vi "DFT_Update Spectra.vi"(6 "averages completed":dbl, 9 "spectra info":T1[](array[typedef]) {"x-axis units" items=["Time (s)"=0, "Frequency-CB (Hz)"=1, "Frequency-CPB (Hz)"=1248, "Frequency-Arbitrary (Hz)"=2357, "Quefrency (s)"=2, "Revolutions (rev)"=3, "Order"=4, "Speed (RPM)"=11, "Speed (rad/s)"=21, "Index"=65535]; "weighting filter" items=["Linear", "A-weighting", "B-weighting", "C-weighting", "ITU-R 468-4", "Dolby", "CCITT", "C-message", "Wb", "Wc", "Wd", "We", "Wf", "Wh", "Wj", "Wk", "Wm", "AES17 20 kHz lowpass", "AES17 40 kHz lowpass", "AES17 20 kHz highpass", "AES17 40 kHz highpass"]; "dB reference [EU]" format="%.2f"; "engineering units" items=["custom..."=0, "V"=1, "A"=21, "C"=30, "pC"=31, "s"=32, "-"=29, "Pa"=2, "N"=20, "g"=3, "m/s^2"=4, "m/s"=5, "m"=6, "mm/s"=12, "mm"=13, "micron/s"=14, "micron"=15, "in/s^2"=7, "in/s"=8, "in"=9, "mil/s"=10, "mil"=11, "rad/s^2"=16, "rad/s"=17, "rad"=18, "deg/s^2"=26, "deg/s"=27, "deg"=28, "RPM"=22, "cycle/s^2"=23, "Hz"=24, "cycle"=25, "strain"=19]; "spectral info"."window" items=["None "=0, "Hanning"=1, "Hamming"=2, "Blackman-Harris"=3, "Exact Blackman"=4, "Blackman"=5, "Flat Top"=6, "4 Term B-Harris "=7, "7 Term B-Harris"=8, "Low Sidelobe"=9, "Force - Exponential"=10, "Gaussian"=62]}, 10 "spectra":cluster{"f0":dbl, "df":dbl, "magnitude":dbl[]}[](array[cluster]) {"magnitude" format="%.2p"; "df" format="%.2p"; "f0" format="%.2p"}, 11 "Data":T7={"First Time"=FALSE, "Show Results Window"=FALSE, "Show Results Window Clicked"=FALSE, "Window"=1, "overlap"=50, "Block Duration"=0.1, "Averaging parameters"={"averaging mode"=enum."No averaging", "weighting mode"=enum."Exponential", "number of averages"=10}, "buffer out"=refnum, "Avg Spectra"=refnum, "Spectra UI"=refnum} {"Averaging parameters"."number of averages" min=1; "Window" items=["Rectangle"=0, "Hanning"=1, "Hamming"=2, "Blackman-Harris"=3, "Exact Blackman"=4, "Blackman"=5, "Flat Top"=6, "4 Term B-Harris "=7, "7 Term B-Harris"=8, "Low Sidelobe"=9, "Blackman Nuttall"=11, "Triangle"=30, "Bartlett-Hanning"=31, "Bohman"=32, "Parzen"=33, "Welch"=34, "Kaiser"=60, "Dolph-Chebyshev"=61, "Gaussian"=62]}) -> (3 "Data out":T7={"First Time"=FALSE, "Show Results Window"=FALSE, "Show Results Window Clicked"=FALSE, "Window"=1, "overlap"=50, "Block Duration"=0.1, "Averaging parameters"={"averaging mode"=enum."No averaging", "weighting mode"=enum."Exponential", "number of averages"=10}, "buffer out"=refnum, "Avg Spectra"=refnum, "Spectra UI"=refnum} {"Averaging parameters"."number of averages" min=1; "Window" items=["Rectangle"=0, "Hanning"=1, "Hamming"=2, "Blackman-Harris"=3, "Exact Blackman"=4, "Blackman"=5, "Flat Top"=6, "4 Term B-Harris "=7, "7 Term B-Harris"=8, "Low Sidelobe"=9, "Blackman Nuttall"=11, "Triangle"=30, "Bartlett-Hanning"=31, "Bohman"=32, "Parzen"=33, "Welch"=34, "Kaiser"=60, "Dolph-Chebyshev"=61, "Gaussian"=62]})   [LabVIEW 2024, in "DFT_Spectra.lvlib" / "DFT_Spectra.lvclass"]
uses:
  DFT_Spectra.lvclass
  DFT_Spectra Data.ctl
  <vilib>/Analysis/4window.llb/windowTd.ctl
  <vilib>/addons/_NISVFA/_Shared subVIs/Data Objects/Waveforms (DBL)/Waveforms (N Ch).lvclass
  <vilib>/addons/_NISVFA/_Shared subVIs/Data Objects/Data/Data.lvclass
  <vilib>/addons/_NISVFA/_Shared subVIs/Controls/svc_Spectrum Info.ctl
  <vilib>/addons/_NISVFA/_Shared subVIs/Controls/svc_X-Axis Units.ctl
  <vilib>/addons/_NISVFA/_Shared subVIs/Controls/svc_Spectrum Type.ctl
  <vilib>/addons/_NISVFA/_Shared subVIs/Controls/svc_Engineering Units Text Ring.ctl
  <vilib>/addons/_NISVFA/_Shared subVIs/Controls/svc_Weighting Filter Text Ring.ctl
  <vilib>/addons/_NISVFA/_Shared subVIs/Controls/svc_Complimentary Spectrum Units.ctl
  <vilib>/addons/_NISVFA/_Shared subVIs/Data Objects/Y (DBL)/Y (N Ch).lvclass/Y (N Ch).ctl
  <vilib>/addons/_NISVFA/_Shared subVIs/Data Objects/Data/Data.lvclass/Data.ctl
  <vilib>/addons/_NISVFA/_Shared subVIs/Data Objects/Y (DBL)/SV Convert Spectra to Data Object.vi
  <vilib>/addons/_NISVFA/_Shared subVIs/Common/sv_Get NI Property Name String.vi
  <vilib>/addons/_NISVFA/_Shared subVIs/Data Objects/Data/Write Data Attributes.vi
  <vilib>/addons/_NISVFA/_Shared subVIs/Data Objects/subVIs/Set Channel Count.vi
  <vilib>/addons/_NISVFA/_Shared subVIs/Data Objects/Data/Read Data Attributes.vi
  <vilib>/addons/_NISVFA/_Shared subVIs/Data Objects/Y (DBL)/Y (N Ch).lvclass
  C:/Program Files/NI/LVAddons/nisvt/1/vi.lib/addons/_NISVFA/_Shared subVIs/Data Objects/Data/Data.lvclass
  <vilib>/addons/_NISVFA/_Shared subVIs/Data Objects/Y (DBL)/Write Channels Array.vi
  <vilib>/addons/_NISVFA/_Shared subVIs/Spectrum Info/sv_Convert Spectrum Info to Variant Attributes.vi
  <vilib>/Analysis/NI_AALPro.lvlib
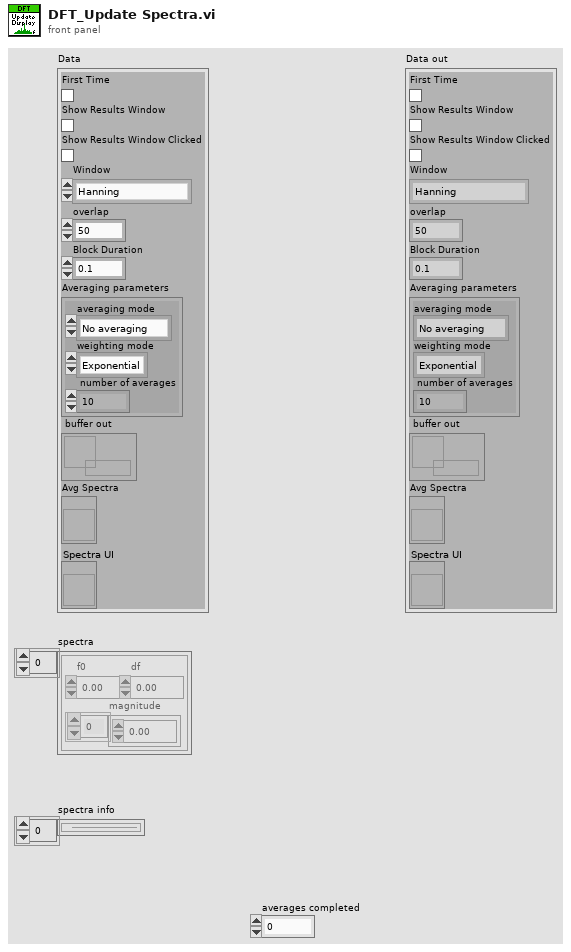
[diagram p1: front panel]
types:
  T1 = typedef "svc_Spectrum Info.ctl" = cluster{"channel name":string, "description":string, "x-axis units":T2, "spectral info":cluster{"spectrum type":T3, "linear/dB":enum16{"linear", "dB"}, "window":u16, "window size":i32, "FFT size":i32}, "engineering units":T4, "custom label":string, "dB reference [EU]":dbl, "peak units":enum16{"rms", "peak", "peak-peak"}, "weighting filter":T5, "spectral density?":bool, "unit label":string, "spectrum skewed?":bool, "complimentary spectrum units":T6}
  T2 = typedef "svc_X-Axis Units.ctl" = u16
  T3 = typedef "svc_Spectrum Type.ctl" = enum16{"FFT Spectrum [complex]", "Amplitude [Magnitude]", "Power [Magnitude^2]", "Cross Spectrum [complex]", "Frequency Response [Complex]"}
  T4 = typedef "svc_Engineering Units Text Ring.ctl" = u16
  T5 = typedef "svc_Weighting Filter Text Ring.ctl" = u16
  T6 = typedef "svc_Complimentary Spectrum Units.ctl" = enum16{"none", "radians", "degrees", "cycles", "imaginary"}
  T7 = typedef "DFT_Spectra.lvlib/DFT_Spectra.lvclass/DFT_Spectra Data.ctl" = cluster{"First Time":bool, "Show Results Window":bool, "Show Results Window Clicked":bool, "Window":T8, "overlap":i32, "Block Duration":dbl, "Averaging parameters":cluster{"averaging mode":enum16{"No averaging", "Vector averaging", "RMS averaging", "Peak hold"}, "weighting mode":enum16{"Linear", "Exponential"}, "number of averages":u32}, "buffer out":refnum<data-value>, "Avg Spectra":refnum<vi>, "Spectra UI":refnum<vi>}
  T8 = typedef "NI_AALPro.lvlib/windowTd.ctl" = u32
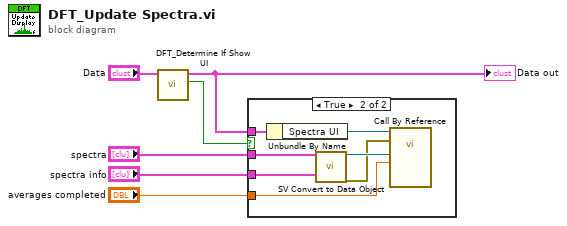
[diagram p0: block diagram]
diagram:
  n1 = call "DFT_Determine If Show UI.vi"("Data"="Data") -> ("Show window"=w3:bool, "Data out"=w4:T7)  [unwired: 9 in]
  "Data out" <- w4
  n2 = case shown="True" w3 {
    tunnel: "averages completed" -> [_ w12]
    tunnel: w4 -> [_ w11]
    tunnel: "spectra" -> [_ w10]
    tunnel: "spectra info" -> [_ w9]
    frame False {
    }
    frame True {
      n3 = Unbundle By Name(w11) -> ("Spectra UI"=w13:refnum<vi>)
      n4 = call-poly <vilib>:"SV Convert to Data Object.vi"("spectra"=w10, "spectra info"=w9) -> ("Spectrum Data"=w8:refnum<class "Data.lvclass">, "error out"=w7:errorcluster)  [unwired: 16 in]
      n5 = call-by-ref "?"(reference=w13, error in=w7, "averages completed"=w12, "Spectrum Data"=w8) -> ()  [unwired: 10 in, 2 out]
    }
  }
